vi "connection handler.vi"(9 "parameters":T1, 10 "websocket standalone server in":refnum<class "websocket standalone server.lvclass">, 11 "connection ID":refnum<k5>) -> ()   [LabVIEW 2013, in "websocket standalone server.lvclass"]
uses:
  websocket standalone server.lvclass
  websocket connection parameters.ctl
  HTTP server/http response.ctl
  HTTP server/http response packet type.ctl
  HTTP headers/http header data.ctl
  websocket data packet.ctl
  websocket message type.ctl
  websocket standalone server.lvclass/websocket standalone server.ctl
  websocket sourced packet.ctl
  <vilib>/dlg_ctls.llb/Space Constant.vi
  <vilib>/Utility/error.llb/Trim Whitespace.vi
  HTTP headers/http headers.lvlib
  HTTP server/Basic HTTP server.lvclass
  websocket core.lvlib
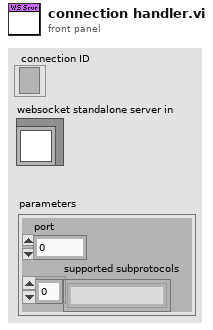
[diagram p1: front panel]
types:
  T1 = typedef "websocket standalone server.lvclass/websocket connection parameters.ctl" = cluster{"port":u16, "supported subprotocols":string[]}
  T2 = enum16{"Standard", "Buffered", "CRLF", "Immediate"}
  T3 = typedef "Basic HTTP server.lvclass/http response.ctl" = cluster{"packet type":T4, "reason code":u16, "status string":string, "headers":T5, "cookies":string[], "data":string}
  T4 = typedef "Basic HTTP server.lvclass/http response packet type.ctl" = enum16{"full response", "header only", "data only", "last data"}
  T5 = typedef "http headers.lvlib/http header data.ctl" = cluster{"fields":string[], "values":string[]}
  T6 = typedef "websocket standalone server.lvclass/websocket data packet.ctl" = cluster{"message type":T7, "data":string}
  T7 = typedef "websocket standalone server.lvclass/websocket message type.ctl" = enum16{"UTF8 data", "binary data", "close", "ping", "pong"}
  T8 = typedef "websocket standalone server.lvclass/websocket sourced packet.ctl" = cluster{"connection":refnum<queue>, "packet":T6}
  T9 = typedef "websocket core.lvlib/first byte header.ctl" = cluster{"fin":bool, "RSRV1":bool, "RSRV2":bool, "RSRV3":bool, "opcode":u8}
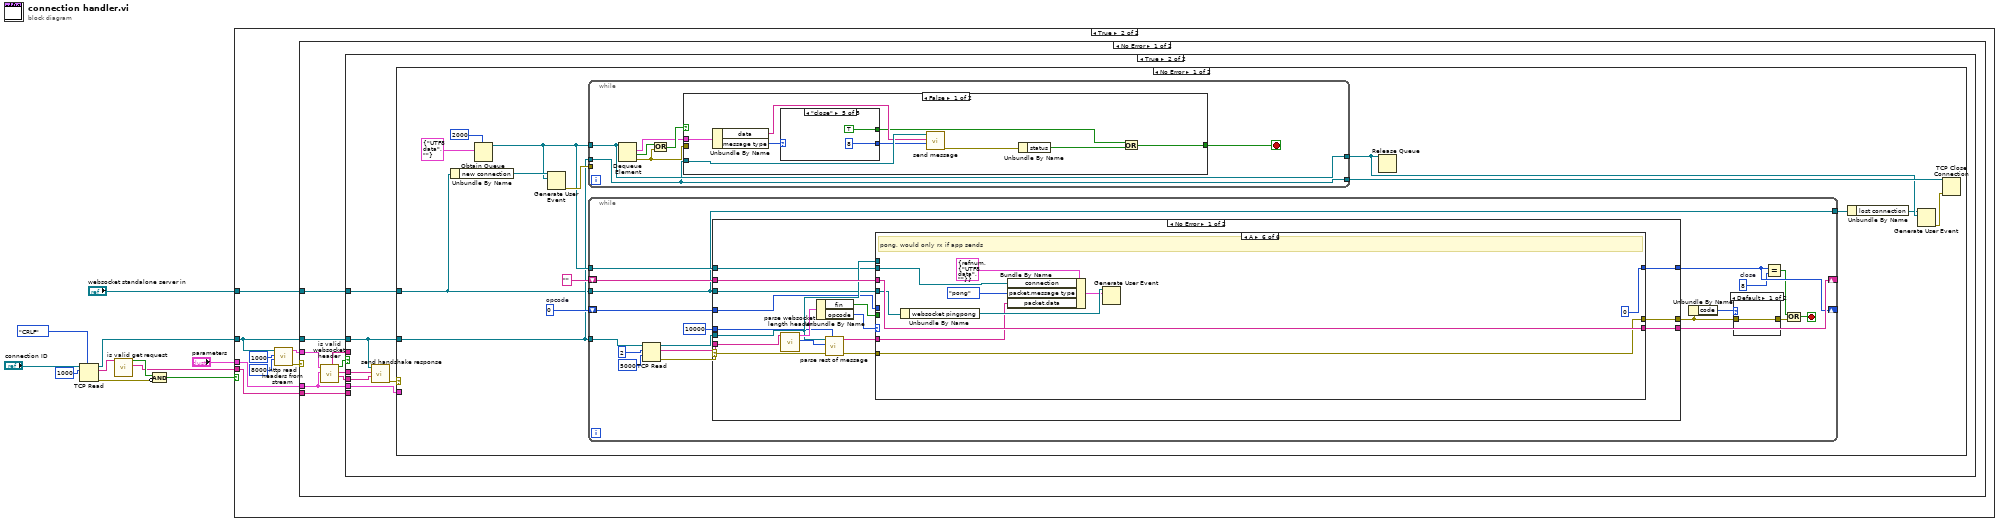
[diagram p0: block diagram]
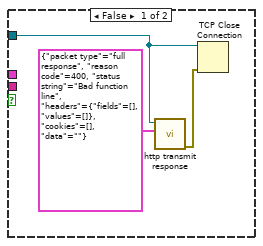
[diagram p2: hidden frame]
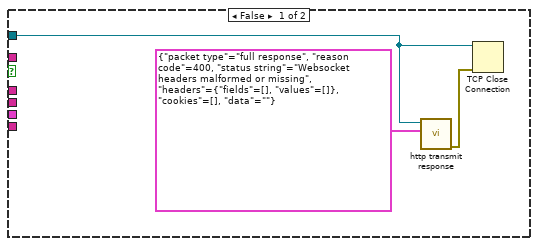
[diagram p3: hidden frame]
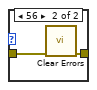
[diagram p4: hidden frame]
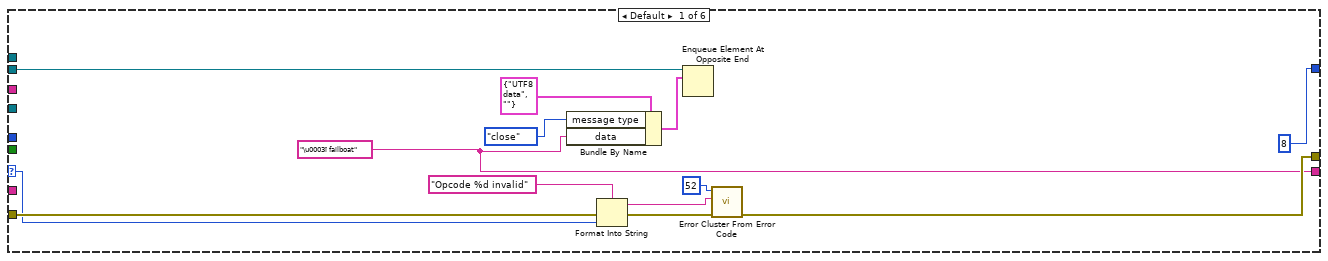
[diagram p5: hidden frame]
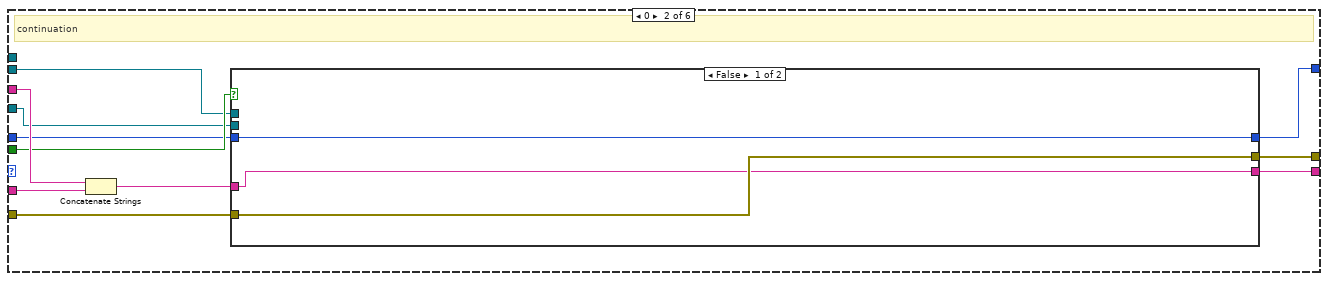
[diagram p6: hidden frame]
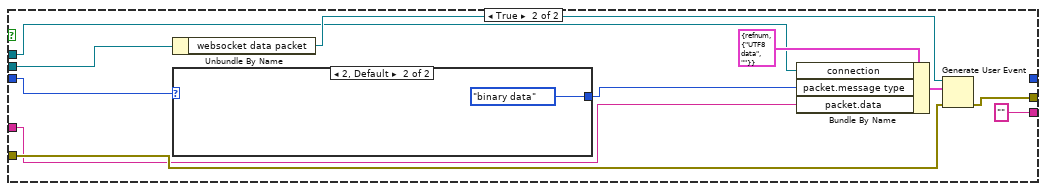
[diagram p7: hidden frame]
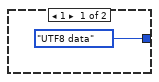
[diagram p8: hidden frame]
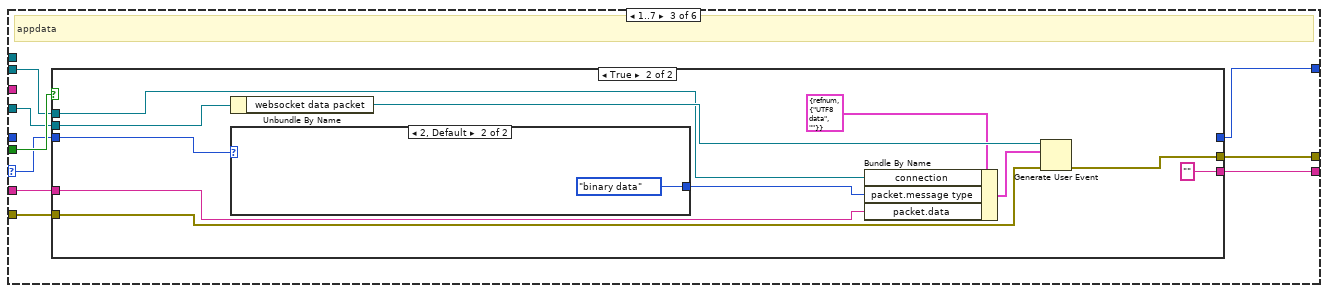
[diagram p9: hidden frame]
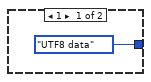
[diagram p11: hidden frame]
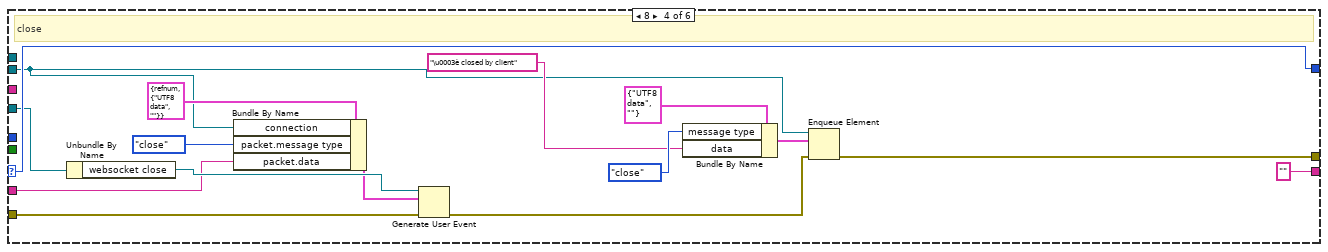
[diagram p12: hidden frame]
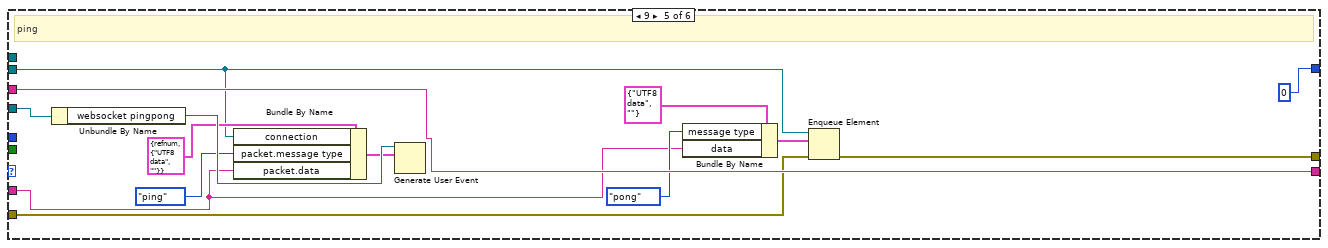
[diagram p13: hidden frame]
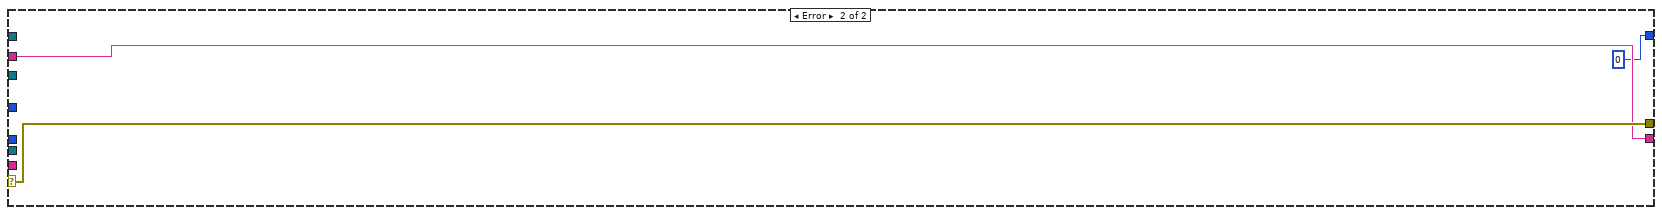
[diagram p14: hidden frame]
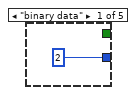
[diagram p15: hidden frame]
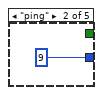
[diagram p16: hidden frame]
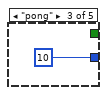
[diagram p17: hidden frame]
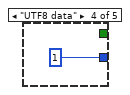
[diagram p18: hidden frame]
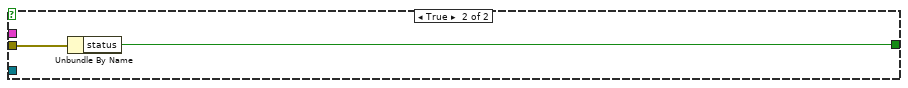
[diagram p19: hidden frame]
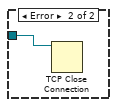
[diagram p20: hidden frame]
diagram:
  n1 = TCP Read(connection ID="connection ID", bytes to read=1000, 7:T2."CRLF" ("mode (standard)")) -> (connection ID out=w4:refnum<k5>, data out=w8:string, error out=w6:errorcluster)  [unwired: 2 in]
  n2 = call "is valid get request.vi"("first line"=w8) -> ("request URI"=w2:string, "valid GET?"=w7:bool)  [unwired: 9 in]
  n3 = Compound Arithmetic op=AND(w7, invert w6) -> (w5:bool)
  n4 = case shown="True" w5 {
    tunnel: w4 -> [w13 w17]
    tunnel: "parameters" -> [_ w18]
    tunnel: w2 -> [_ w16]
    tunnel: "websocket standalone server in" -> [_ w15]
    frame False {
      n5 = call "http transmit response.vi"("application request"=T3 {"packet type"=enum."full response", "reason code"=400, "status string"="Bad function line", "headers"={"fields"=[], "values"=[]}, "cookies"=[], "data"=""}, "tcp connection"=w13) -> ("error out"=w14:errorcluster)  [unwired: 9 in]
      n6 = TCP Close Connection(connection ID=w13, error in (no error)=w14) -> ()  [unwired: 1 in, 2 out]
    }
    frame True {
      n7 = call "http read headers from stream.vi"("max header size"=8000, "timeout ms"=1000, "TCP Network Connection in"=w17) -> ("error out"=w19:errorcluster, "headers"=w20:T5)  [unwired: 7 in]
      n8 = case shown="No Error" w19 {
        tunnel: w20 -> [w31 _]
        tunnel: w18 -> [w24 _]
        tunnel: w17 -> [w29 w227]
        tunnel: w16 -> [w25 _]
        tunnel: w15 -> [w23 _]
        frame No Error {
          n9 = call "is valid websocket header.vi"("parameters"=w24, "headers"=w31) -> ("supported protocols"=w27:string[], "return sec key"=w28:string, "valid websocket headers"=w30:bool, "host field"=w26:string)  [unwired: 6 in]
          n10 = case shown="True" w30 {
            tunnel: w29 -> [w32 w39]
            tunnel: w28 -> [_ w38]
            tunnel: w27 -> [_ w37]
            tunnel: w26 -> [_ _]
            tunnel: w25 -> [_ _]
            tunnel: w24 -> [_ w36]
            tunnel: w23 -> [_ w35]
            frame False {
              n11 = call "http transmit response.vi"("application request"=T3 {"packet type"=enum."full response", "reason code"=400, "status string"="Websocket headers malformed or missing", "headers"={"fields"=[], "values"=[]}, "cookies"=[], "data"=""}, "tcp connection"=w32) -> ("error out"=w34:errorcluster)  [unwired: 9 in]
              n12 = TCP Close Connection(connection ID=w32, error in (no error)=w34) -> ()  [unwired: 1 in, 2 out]
            }
            frame True {
              n13 = call "send handshake response.vi"("supported protocols"=w37, "return sec key"=w38, "TCP Network Connection in"=w39) -> ("error out"=w40:errorcluster)  [unwired: 8 in]
              n14 = case shown="No Error" w40 {
                tunnel: w39 -> [w45 w226]
                tunnel: w36 -> [_ _]
                tunnel: w35 -> [w44 _]
                frame No Error {
                  w46 = u8 0  # opcode
                  n15 = Unbundle By Name(w44) -> ("new connection"=w49:refnum<user-event>)
                  n16 = Obtain Queue(max queue size (-1, unlimited)=2000, element data type=T6 {"message type"=enum."UTF8 data", "data"=""} ("packet")) -> (queue out=w47:refnum<queue>)  [unwired: 3 in, 2 out]
                  n17 = Generate User Event(user event=w49, event data cluster=w47) -> (error out=w50:errorcluster)  [unwired: 2 in, 1 out]
                  n18 = while {
                    tunnel: w47 -> [w203]
                    tunnel: w45 -> [w202]
                    tunnel: [w203] -> w51
                    tunnel: [w202] -> w52
                    tunnel: w50 -> [_]
                    stop <- w206 stop-if-true
                    n19 = Dequeue Element(queue=w203) -> (element=w204:T6, timed out?=w208:bool, error out=w205:errorcluster)  [unwired: 2 in, 1 out]
                    n20 = Or(x=w208, y=w205) -> (x .or. y?=w207:bool)
                    n21 = case shown="False" w207 {
                      tunnel: [w210 w224] -> w206
                      tunnel: w205 -> [_ w225]
                      tunnel: w204 -> [w216 _]
                      tunnel: w202 -> [w217 _]
                      frame False {
                        n22 = Unbundle By Name(w216) -> ("data"=w213:string, "message type"=w212:T7)
                        n23 = case shown="\"close\"" w212 {
                          tunnel: [u8 2 ("opcode") u8 9 ("opcode") u8 10 ("opcode") u8 1 ("opcode") u8 8 ("opcode")] -> w211
                          tunnel: [_ _ _ _ TRUE] -> w209
                          frame "binary data" {
                          }
                          frame "ping" {
                          }
                          frame "pong" {
                          }
                          frame "UTF8 data" {
                          }
                          frame "close" {
                          }
                        }
                        n24 = call "send message.vi"("opcode"=w211, "data"=w213, "TCP Network Connection in"=w217) -> ("error out"=w215:errorcluster)  [unwired: 8 in]
                        n25 = Unbundle By Name(w215) -> ("status"=w214:bool)
                        n26 = Or(x=w209, y=w214) -> (x .or. y?=w210:bool)
                      }
                      frame True {
                        n27 = Unbundle By Name(w225) -> ("status"=w224:bool)
                      }
                    }
                  }
                  n28 = while {
                    shift-right: [w70] -> _
                    shift-left: "" -> [w71]
                    tunnel: w47 -> [w64]
                    tunnel: w44 -> [w57]
                    shift-right: [w60] -> _
                    shift-left: w46 -> [w63]
                    tunnel: w45 -> [w62]
                    tunnel: [w57] -> w43
                    stop <- w61 stop-if-true
                    w59 = u8 8  # close
                    n29 = TCP Read(connection ID=w62, bytes to read=2, 9:5000 ("base timeout (5000)")) -> (connection ID out=w67:refnum<k5>, data out=w69:string, error out=w66:errorcluster)  [unwired: 2 in]
                    n30 = case shown="No Error" w66 {
                      selector: w66 -> [w93 w201]
                      tunnel: w69 -> [w92 _]
                      tunnel: w67 -> [w82 _]
                      tunnel: [w89 w201] -> w56
                      tunnel: w71 -> [w85 w200]
                      tunnel: [w86 w200] -> w70
                      tunnel: 10000 ("continuation timeout (10000)") -> [w81 _]
                      tunnel: w64 -> [w80 _]
                      tunnel: w57 -> [w79 _]
                      tunnel: w63 -> [w78 _]
                      tunnel: [w77 u8 0 ("opcode")] -> w60
                      frame No Error {
                        n31 = call "parse websocket length header.vi"("header string"=w92) -> ("mask(1)+length(7)"=w91:u8, "first byte"=w90:T9)  [unwired: 9 in]
                        n32 = Unbundle By Name(w90) -> ("fin"=w83:bool, "opcode"=w87:u8)
                        n33 = call "parse rest of message.vi"("continuation timeout ms (2000)"=w81, "error in"=w93, "mask(1)+length(7)"=w91, "TCP Network Connection in"=w82) -> ("error out"=w88:errorcluster, "unmasked data"=w84:string)  [unwired: 6 in]
                        n34 = case shown="A" w87 {
                          selector: w87 -> [w101 _ w134 w174 _ _]
                          tunnel: [w105 w114 w135 w170 w182 w197] -> w89
                          tunnel: w88 -> [w106 w113 w136 w164 w187 w197]
                          tunnel: [w96 w111 w141 "" ("unmasked data") w188 w198] -> w86
                          tunnel: w85 -> [_ w117 _ _ w188 w198]
                          tunnel: w84 -> [_ w116 w142 w160 w175 w190]
                          tunnel: w83 -> [_ w115 w140 _ _ _]
                          tunnel: w82 -> [_ _ _ _ _ _]
                          tunnel: w80 -> [w99 w109 w138 w161 w176 w189]
                          tunnel: w79 -> [_ w110 w137 w162 w181 w191]
                          tunnel: w78 -> [_ w108 _ _ _ _]
                          tunnel: [u8 8 ("opcode") w107 w139 w174 u8 0 ("opcode") u8 0 ("opcode")] -> w77
                          frame Default {
                            w96 = "\u0003ï failboat" ("data")
                            n35 = Bundle By Name(cluster=T6 {"message type"=enum."UTF8 data", "data"=""} ("element"), "message type"=websocket_message_type."close", "data"=w96) -> (w97:T6)
                            n36 = Format Into String(format string="Opcode %d invalid", error in=w106, w101) -> (resulting string=w102:string, error out=w103:errorcluster)  [unwired: 1 in]
                            n37 = Enqueue Element At Opposite End(queue=w99, element=w97) -> ()  [unwired: 2 in, 3 out]
                            n38 = call <vilib>:"Error Cluster From Error Code.vi"("error in (no error)"=w103, "error message (\"\")"=w102, "error code (0)"=52) -> ("error out"=w105:errorcluster)  [unwired: 6 in]
                          }
                          frame 0 {
                            # "continuation"
                            n39 = Concatenate Strings(w117, w116) -> (w112:string)
                            n40 = case shown="False" w115 {
                              tunnel: [w120 w131] -> w114
                              tunnel: w113 -> [w120 w130]
                              tunnel: w112 -> [w119 w122]
                              tunnel: [w119 ""] -> w111
                              tunnel: w110 -> [_ w129]
                              tunnel: w109 -> [_ w125]
                              tunnel: w108 -> [w118 w124]
                              tunnel: [w118 _] -> w107
                              frame False {
                              }
                              frame True {
                                n41 = Unbundle By Name(w129) -> ("websocket data packet"=w128:refnum<user-event>)
                                n42 = case shown="2, Default" w124 {
                                tunnel: [websocket_message_type."UTF8 data" ("packet.message type") websocket_message_type."binary data" ("packet.message type")] -> w123
                                frame 1 {
                                }
                                frame 2, Default {
                                }
                                }
                                n43 = Bundle By Name(cluster=T8 {"connection"=refnum, "packet"={"message type"=enum."UTF8 data", "data"=""}} ("event data"), "connection"=w125, "packet.message type"=w123, "packet.data"=w122) -> (w126:T8)
                                n44 = Generate User Event(user event=w128, event data cluster=w126, error in=w130) -> (error out=w131:errorcluster)  [unwired: 1 in, 1 out]
                              }
                            }
                          }
                          frame 1..7 {
                            # "appdata"
                            n45 = case shown="True" w140 {
                              tunnel: [w145 w156] -> w135
                              tunnel: w136 -> [w145 w155]
                              tunnel: w142 -> [w144 w147]
                              tunnel: [w144 ""] -> w141
                              tunnel: w137 -> [_ w154]
                              tunnel: w138 -> [_ w150]
                              tunnel: w134 -> [w143 w149]
                              tunnel: [w143 _] -> w139
                              frame False {
                              }
                              frame True {
                                n46 = Unbundle By Name(w154) -> ("websocket data packet"=w153:refnum<user-event>)
                                n47 = case shown="2, Default" w149 {
                                tunnel: [websocket_message_type."UTF8 data" ("packet.message type") websocket_message_type."binary data" ("packet.message type")] -> w148
                                frame 1 {
                                }
                                frame 2, Default {
                                }
                                }
                                n48 = Bundle By Name(cluster=T8 {"connection"=refnum, "packet"={"message type"=enum."UTF8 data", "data"=""}} ("event data"), "connection"=w150, "packet.message type"=w148, "packet.data"=w147) -> (w151:T8)
                                n49 = Generate User Event(user event=w153, event data cluster=w151, error in=w155) -> (error out=w156:errorcluster)  [unwired: 1 in, 1 out]
                              }
                            }
                          }
                          frame 8 {
                            # "close"
                            n50 = Unbundle By Name(w162) -> ("websocket close"=w168:refnum<user-event>)
                            n51 = Bundle By Name(cluster=T8 {"connection"=refnum, "packet"={"message type"=enum."UTF8 data", "data"=""}} ("event data"), "connection"=w161, "packet.message type"=websocket_message_type."close", "packet.data"=w160) -> (w166:T8)
                            n52 = Generate User Event(user event=w168, event data cluster=w166, error in=w164) -> (error out=w163:errorcluster)  [unwired: 1 in, 1 out]
                            n53 = Bundle By Name(cluster=T6 {"message type"=enum."UTF8 data", "data"=""} ("element"), "message type"=websocket_message_type."close", "data"="\u0003è closed by client") -> (w172:T6)
                            n54 = Enqueue Element(queue=w161, element=w172, error in (no error)=w163) -> (error out=w170:errorcluster)  [unwired: 1 in, 2 out]
                          }
                          frame 9 {
                            # "ping"
                            n55 = Unbundle By Name(w181) -> ("websocket pingpong"=w180:refnum<user-event>)
                            n56 = Bundle By Name(cluster=T8 {"connection"=refnum, "packet"={"message type"=enum."UTF8 data", "data"=""}} ("event data"), "connection"=w176, "packet.message type"=websocket_message_type."ping", "packet.data"=w175) -> (w178:T8)
                            n57 = Generate User Event(user event=w180, event data cluster=w178) -> ()  [unwired: 2 in, 2 out]
                            n58 = Bundle By Name(cluster=T6 {"message type"=enum."UTF8 data", "data"=""} ("element"), "message type"=websocket_message_type."pong", "data"=w175) -> (w184:T6)
                            n59 = Enqueue Element(queue=w176, element=w184, error in (no error)=w187) -> (error out=w182:errorcluster)  [unwired: 1 in, 2 out]
                          }
                          frame 10 {
                            # "pong, would only rx if app sends"
                            n60 = Unbundle By Name(w191) -> ("websocket pingpong"=w195:refnum<user-event>)
                            n61 = Bundle By Name(cluster=T8 {"connection"=refnum, "packet"={"message type"=enum."UTF8 data", "data"=""}} ("event data"), "connection"=w189, "packet.message type"=websocket_message_type."pong", "packet.data"=w190) -> (w193:T8)
                            n62 = Generate User Event(user event=w195, event data cluster=w193) -> ()  [unwired: 2 in, 2 out]
                          }
                        }
                      }
                      frame Error {
                      }
                    }
                    n63 = Unbundle By Name(w56) -> ("code"=w55:i32)
                    n64 = case shown="Default" w55 {
                      tunnel: w56 -> [w74 w76]
                      tunnel: [w74 w75] -> w65
                      frame Default {
                      }
                      frame 56 {
                        n65 = call <vilib>:"Clear Errors.vi"("error in (no error)"=w76) -> ("error out"=w75:errorcluster)  [unwired: 6 in]
                      }
                    }
                    n66 = Equal?(x=w60, y=w59) -> (x = y?=w58:bool)
                    n67 = Or(x=w58, y=w65) -> (x .or. y?=w61:bool)
                  }
                  n68 = Release Queue(queue=w51) -> ()  [unwired: 2 in, 3 out]
                  n69 = Unbundle By Name(w43) -> ("lost connection"=w42:refnum<user-event>)
                  n70 = Generate User Event(user event=w42, event data cluster=w51) -> (error out=w41:errorcluster)  [unwired: 2 in, 1 out]
                  n71 = TCP Close Connection(connection ID=w52, error in (no error)=w41) -> ()  [unwired: 1 in, 2 out]
                }
                frame Error {
                  n72 = TCP Close Connection(connection ID=w226) -> ()  [unwired: 2 in, 2 out]
                }
              }
            }
          }
        }
        frame Error {
          n73 = call "http transmit response.vi"("application request"=T3 {"packet type"=enum."full response", "reason code"=400, "status string"="Bad headers", "headers"={"fields"=[], "values"=[]}, "cookies"=[], "data"=""}, "tcp connection"=w227) -> ("error out"=w229:errorcluster)  [unwired: 9 in]
          n74 = TCP Close Connection(connection ID=w227, error in (no error)=w229) -> ()  [unwired: 1 in, 2 out]
        }
      }
    }
  }
